vi "Create Known Hosts File.vi"(8 "error in (no error)":errorcluster, 11 "Server Fixture in":refnum<class "Server Fixture.lvclass">) -> (0 "error out":errorcluster, 3 "Server Fixture out":refnum<class "Server Fixture.lvclass">)   [LabVIEW 2013, in "libssh2_integration_tests.lvlib" / "Server Fixture.lvclass"]
uses:
  Server Fixture.lvclass
  Server Fixture.lvclass/Server Fixture.ctl
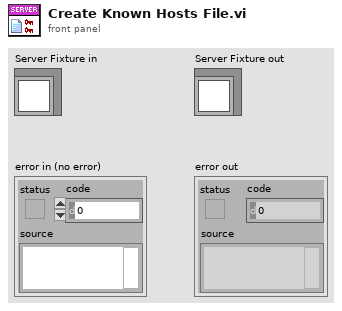
[diagram p1: front panel]
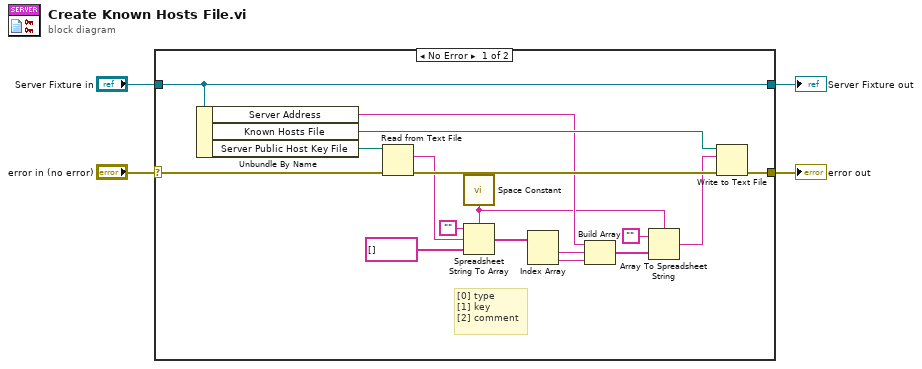
[diagram p0: block diagram]
diagram:
  n1 = case shown="No Error" "error in (no error)" {
    selector: "error in (no error)" -> [w21 w23]
    tunnel: [w14 w23] -> w3
    tunnel: [w20 w22] -> w1
    tunnel: "Server Fixture in" -> [w20 w22]
    frame No Error {
      # "[0] type\n[1] key\n[2] comment"
      n2 = Unbundle By Name(w20) -> ("Server Address"=w9:string, "Known Hosts File"=w13:path, "Server Public Host Key File"=w18:path)
      n3 = Read from Text File(file (use dialog)=w18, error in=w21) -> (text=w17:string, error out=w19:errorcluster)  [unwired: 2 in, 2 out]
      n4 = call <vilib>:"Space Constant.vi"() -> ("String"=w7:string)
      n5 = Spreadsheet String To Array(delimiter (Tab)=w7, format string="", spreadsheet string=w17, array type (2D Dbl)=string[] []) -> (array=w12:string[])
      n6 = Index Array(array=w12) -> (element #1=w11:string, element #2=w10:string)  [unwired: 2 in]
      n7 = Build Array(w9, w11, w10) -> (w8:string[])
      n8 = Array To Spreadsheet String(delimiter (Tab)=w7, array=w8, 3:"") -> (spreadsheet string=w6:string)
      n9 = Write to Text File(file (use dialog)=w13, text=w6, error in=w19) -> (error out=w14:errorcluster)  [unwired: 1 in, 2 out]
    }
    frame Error {
    }
  }
  "error out" <- w3
  "Server Fixture out" <- w1
